vi "CSM Critical Error.vi"(8 "error in (no error)":errorcluster, 10 "Arugments (As Reason)":string, 11 "CSM Name":string) -> (0 "error out":errorcluster)   [LabVIEW 2017, in "Communicable State Machine.lvlib"]
doc: "Generates an error cluster describing a CSM Critical Error. A Critical Error is a severe error occurring within the CSM framework that cannot be handled or replied to by user code. A common cause is a duplicate module name.\n\n-- <b>Controls</b> --\n- <b>CSM Name</b>: CSM module name.\n- <b>Arguments (As Reason)</b>: Reason for the error."
uses:
  Communicable State Machine.lvlib
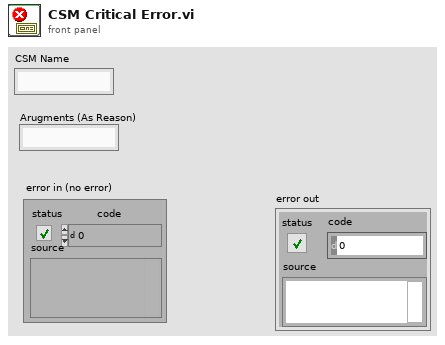
[diagram p1: front panel]
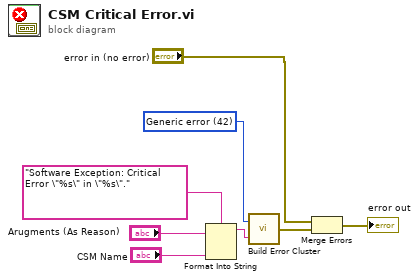
[diagram p0: block diagram]
diagram:
  w5 = 42 items=["No error", "Argument error", "Memory is full", "Out of zone", "End of file", "File already open", "Generic file I/O error", "File not found", "File permission error", "Disk is full", "Duplicate path", "Too many files open", "System feature not enabled", "Resource file not found", "Cannot add resource", "Resource not found", "Image not found", "Image memory error", "Pen does not exist", "Config type invalid", "Config token not found", "Config parse error", "Config memory error", "Bad external code format", "Bad external code offset", "External code not present", "Null window", "Destroy window error", "Null menu", "Print aborted", "Bad print record", "Print driver error", "Windows error during printing", "Memory error during printing", "Print dialog error", "Generic print error", "Invalid device refnum", "Device not found", "Device parameter error", "Device unit error", "Cannot open device", "Device call aborted", "Generic error", "Cancelled by user", "Object ID too low", "Object ID too high", "Object not in heap", "Unknown heap", "Unknown object (invalid DefProc)", "Unknown object (DefProc not in table)", "Message out of range", "Invalid (null) method", "Unknown message", "Manager call not supported", "Bad address", "Network operation in progress", "Network operation timed out", "Connection is busy", "Network attribute not supported", "Network error", "Address in use", "System out of memory", "Connection aborted", "Connection refused", "Not connected", "Already connected", "Connection closed", "Initialization error (interapplication manager)", "Bad occurrence", "Wait on unbound occurrence handler", "Occurrence queue overflow", "Datalog type conflict", "Unused", "Unrecognized type (interapplication manager)", "Memory corrupt", "Failed to make temporary DLL", "Old CIN version", "Drag socket not found", "Failed to load drop-object", "Failed to register OLE object", "Failed to release OLE object", "Format specifier type mismatch", "Unknown format specifier", "Too few format specifiers", "Too many format specifiers", "Scan failed", "Newer CIN version", "Error converting to variant", "Runtime menu error", "Password tampered", "Variant attribute not found", "Incompatible variant data type", "Event data is not available", "Event Store is not present", "Occurrence is not found", "Event Queue is not created", "Event info is not available", "Refnum passed is NULL", "Error retrieving Class GUID", "Error retrieving CoClass GUID", "Error retrieving TypeLib GUID.", "Bad built application magic bytes.", "Specific driver is different from the specific driver associated with the Logical Name.", "There is no session opened to the class driver.", "Max Error", "MAX - Error with config objects", "MAX - Error loading configuration", "MAX - Group not supported"]
  n1 = Format Into String(format string="Software Exception: Critical Error \"%s\" in \"%s\"." ("message"), "Arugments (As Reason)", "CSM Name") -> (resulting string=w6:string)  [unwired: 2 in, 1 out]
  n2 = call "Build Error Cluster.vi"("String to Prepend to Source (\"\")"=w6, "Code"=w5) -> ("error out"=w7:errorcluster)
  n3 = Merge Errors("error in (no error)", w7) -> (→"error out":errorcluster)
